vi "KeithleyRange.vi"(8 "error in":errorcluster, 9 "Range (V)/Auto(0)":dbl, 10 "address (16)":i16=16, 11 "bus (0)":i32) -> (0 "error out":errorcluster)   [LabVIEW 2017]
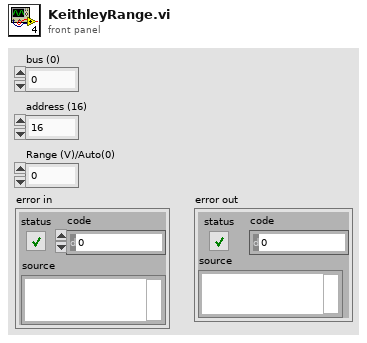
[diagram p1: front panel]
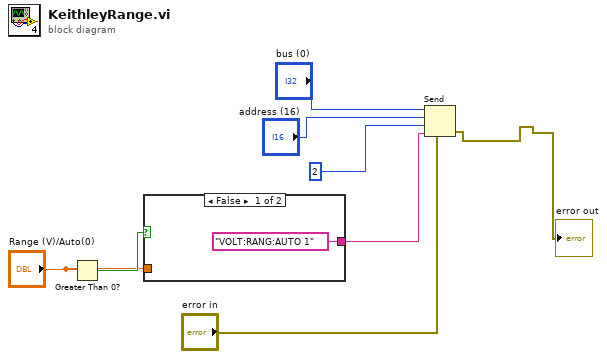
[diagram p0: block diagram]
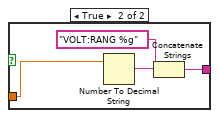
[diagram p2: hidden frame]
diagram:
  n1 = Greater Than 0?(x="Range (V)/Auto(0)") -> (x > 0?=w3:bool)
  n2 = case shown="False" w3 {
    tunnel: ["VOLT:RANG:AUTO 1" w11] -> w8
    tunnel: "Range (V)/Auto(0)" -> [_ w10]
    frame False {
    }
    frame True {
      n3 = Number To Decimal String(number=w10) -> (decimal integer string=w13:string)  [unwired: 1 in]
      n4 = Concatenate Strings("VOLT:RANG %g", w13) -> (w11:string)
    }
  }
  n5 = Send(0:"bus (0)", 2:"address (16)", 3:i16 2 ("mode"), 4:"error in", 5:w8) -> (8:→"error out":errorcluster)  [unwired: 2 out]
